vi "Set Item Type.vi"(8 "error in (no error)":errorcluster, 10 "DNL_Type":T1=enum."New VI", 11 "ClickableText in":refnum<class "ClickableText.lvclass">) -> (0 "error out":errorcluster, 3 "ClickableText out":refnum<class "ClickableText.lvclass">)   [LabVIEW 2009, in "NavScreen.lvlib" / "ClickableText.lvclass"]
uses:
  ClickableText.lvclass
  ItemData_Type.ctl
  ClickableText.lvclass/ClickableText.ctl
  NavScreen.lvlib
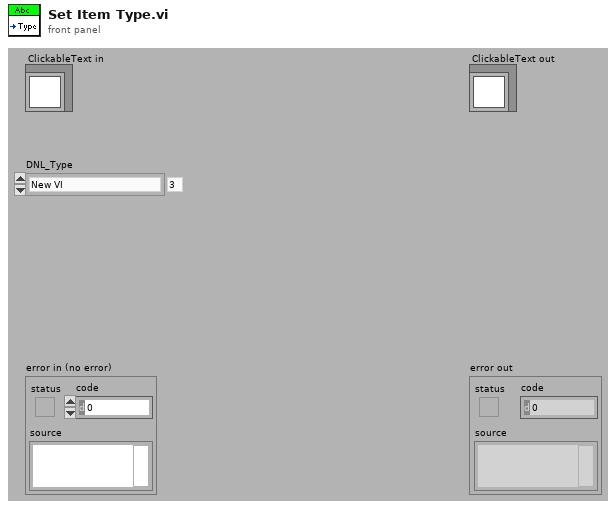
[diagram p1: front panel]
types:
  T1 = typedef "NavScreen.lvlib/ItemData_Type.ctl" = enum16{"None", "Folder", "New Project", "New VI", "Find", "VI", "Project", "New from template", "RT Project Wizard", "PDA Project Wizard", "Control", "Library", "Class", "XControl", "Runtime menu"}
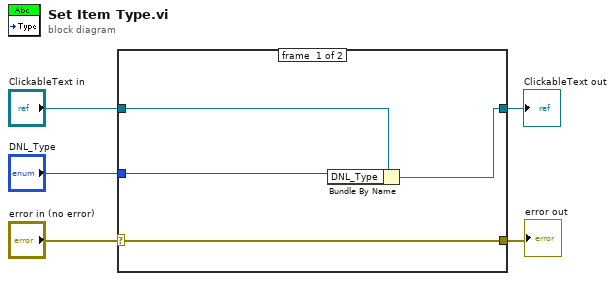
[diagram p0: block diagram]
diagram:
  n1 = case shown="No Error" "error in (no error)" {
    selector: "error in (no error)" -> [w9 w11]
    tunnel: [w9 w11] -> w4
    tunnel: [w6 w10] -> w2
    tunnel: "ClickableText in" -> [w8 w10]
    tunnel: "DNL_Type" -> [w7 _]
    frame #0 {
      n2 = Bundle By Name(cluster=w8, "DNL_Type"=w7) -> (w6:refnum<class "ClickableText.lvclass">)
    }
    frame #1 {
    }
  }
  "error out" <- w4
  "ClickableText out" <- w2
